vi "Get ExternalTemp.vi"(8 "error in (no error)":errorcluster, 11 "VISA resource name":refnum<visa-resource-name>) -> (0 "error out":errorcluster, 1 "ExternalTemp (out)":dbl, 3 "VISA resource name out":refnum<visa-resource-name>, 4 "Is Sensor connected?":bool)   [LabVIEW 2018, in "JULABO DeviceDriver.lvlib"]
doc: "This VI returns the actual temperature value measured by the external sensor.\n\nNote:\nThis function is not available for devices which do not have an external sensor plug."
uses:
  JULABO DeviceDriver.lvlib
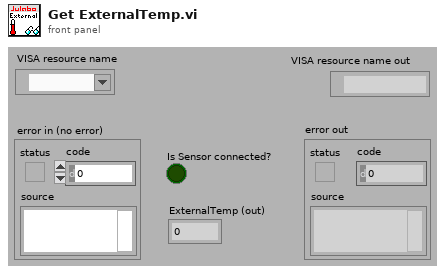
[diagram p1: front panel]
types:
  T1 = typedef "JULABO DeviceDriver.lvlib/InstrumentType.ctl" = enum8{"Default", "FC-Series", "HT30/HT60", "LC4"}
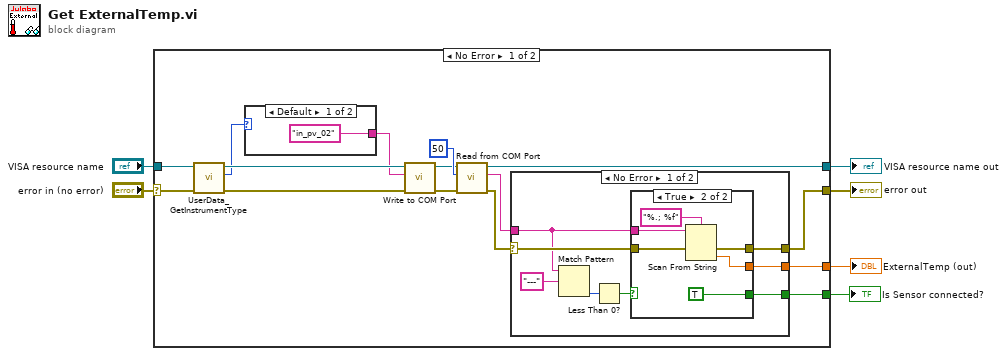
[diagram p0: block diagram]
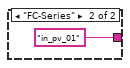
[diagram p2: hidden frame]
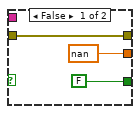
[diagram p3: hidden frame]
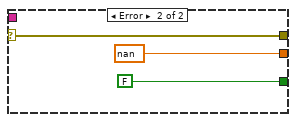
[diagram p4: hidden frame]
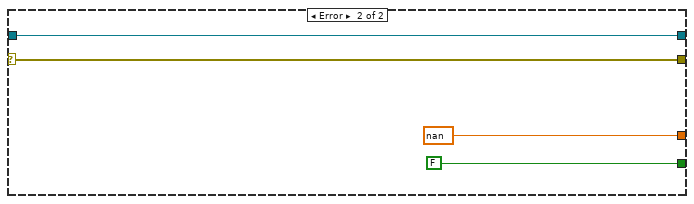
[diagram p5: hidden frame]
diagram:
  n1 = case shown="No Error" "error in (no error)" {
    selector: "error in (no error)" -> [w9 w46]
    tunnel: "VISA resource name" -> [w10 w47]
    tunnel: [w21 w46] -> w4
    tunnel: [w20 w47] -> w3
    tunnel: [w19 nan] -> w2
    tunnel: [w18 FALSE] -> w1
    frame No Error {
      n2 = call "UserData_GetInstrumentType.vi"("Fehler (Eingang)"=w9, "VISA resource name in"=w10) -> ("Fehler (Ausgang)"=w13:errorcluster, "InstrumentType"=w12:T1, "VISA resource name out"=w14:refnum<visa-resource-name>)  [unwired: 3 in]
      n3 = case shown="Default" w12 {
        tunnel: ["in_pv_02" "in_pv_01"] -> w11
        frame Default {
        }
        frame "FC-Series" {
        }
      }
      n4 = call "Write to COM Port.vi"("error in"=w13, "Command (input)"=w11, "VISA resource name in"=w14) -> ("error out"=w7:errorcluster, "VISA resource name out"=w8:refnum<visa-resource-name>)  [unwired: 7 in]
      n5 = call "Read from COM Port.vi"("error in"=w7, "Byte to Read (-1:All)"=50 ("Anzahl der Byte"), "VISA resource name in"=w8) -> ("error out"=w15:errorcluster, "String (output)"=w16:string, "VISA resource name out"=w20:refnum<visa-resource-name>)  [unwired: 5 in, 1 out]
      n6 = case shown="No Error" w15 {
        selector: w15 -> [w31 w43]
        tunnel: w16 -> [w29 _]
        tunnel: [w27 w43] -> w21
        tunnel: [w26 nan] -> w19
        tunnel: [w24 FALSE] -> w18
        frame No Error {
          n7 = Match Pattern(string=w29, regular expression="---") -> (offset past match=w28:i32)  [unwired: 1 in, 3 out]
          n8 = Less Than 0?(x=w28) -> (x < 0?=w25:bool)
          n9 = case shown="True" w25 {
            tunnel: w31 -> [w32 w39]
            tunnel: w29 -> [_ w38]
            tunnel: [w32 w37] -> w27
            tunnel: [nan w36] -> w26
            tunnel: [FALSE TRUE] -> w24
            frame False {
            }
            frame True {
              n10 = Scan From String(format string="%.; %f" ("Format-String"), input string=w38, error in=w39) -> (error out=w37:errorcluster, output 1=w36:dbl)  [unwired: 2 in, 2 out]
            }
          }
        }
        frame Error {
        }
      }
    }
    frame Error {
    }
  }
  "error out" <- w4
  "VISA resource name out" <- w3
  "ExternalTemp (out)" <- w2
  "Is Sensor connected?" <- w1
